vi "GetDigitalInputVals.vi"(8 "error in (no error)":errorcluster, 11 "SerialPortRef":T1) -> (0 "error out":errorcluster, 2 "32 bit array":bool[](array[boolean]), 3 "SerialPortRef 2":T1)   [LabVIEW 2015]
uses:
  <vilib>/Rock Robotics/WPI/SerialPort/WPI_SerialPortRef.ctl
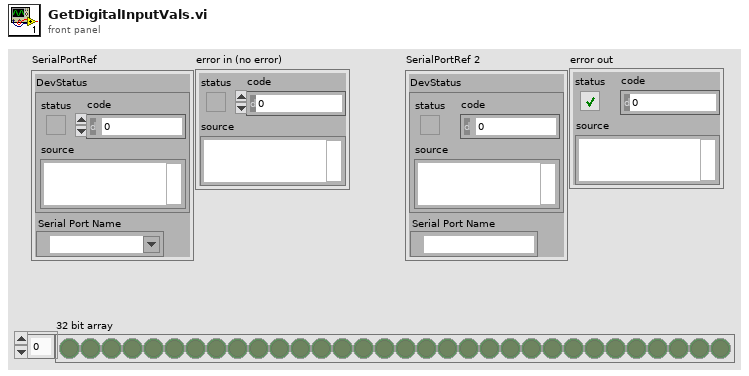
[diagram p1: front panel]
types:
  T1 = typedef "WPI_SerialPortRef.ctl" = cluster{"DevStatus":errorcluster, "Serial Port Name":refnum<visa-resource-name>}
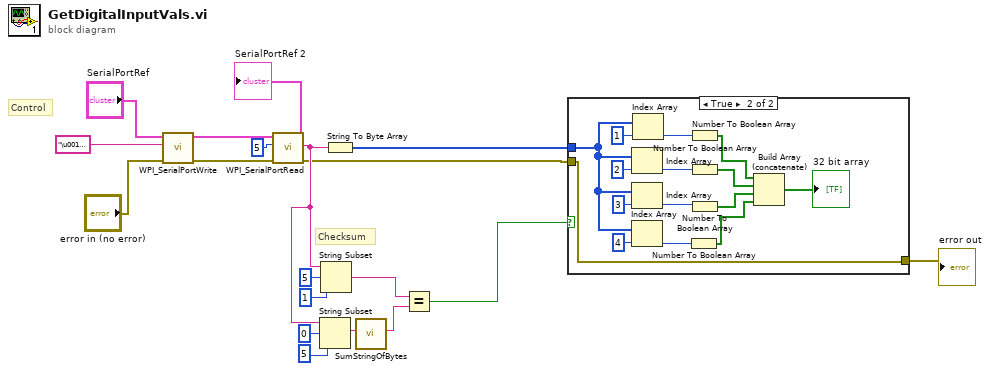
[diagram p0: block diagram]
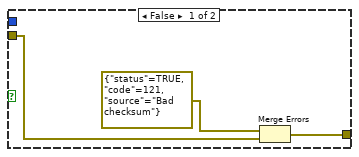
[diagram p2: hidden frame]
diagram:
  # "Checksum"
  # "Control"
  n1 = call <vilib>:"WPI_SerialPortWrite.vi"("error in (no error)"="error in (no error)", "Buffer"="\u0010\u0010", "SerialPortRef"="SerialPortRef") -> ("error out"=w15:errorcluster, "SerialPortRef"=w16:T1)  [unwired: 6 in, 1 out]
  n2 = call <vilib>:"WPI_SerialPortRead.vi"("error in (no error)"=w15, "Num Bytes to Read"=u32 5, "SerialPortRef"=w16) -> ("error out"=w3:errorcluster, "Buffer"=w9:string, "SerialPortRef"=→"SerialPortRef 2":T1)  [unwired: 6 in]
  n3 = String Subset(string=w9, offset (0)=0, length (rest)=5 ("length (rest)")) -> (substring=w6:string)
  n4 = String Subset(string=w9, offset (0)=5, length (rest)=1 ("length (rest)")) -> (substring=w5:string)
  n5 = String To Byte Array(string=w9) -> (unsigned byte array=w12:u8[])
  n6 = call "SumStringOfBytes.vi"("String Of Bytes"=w6) -> ("SumAsString"=w4:string)  [unwired: 10 in]
  n7 = Equal?(x=w5, y=w4) -> (x = y?=w2:bool)
  n8 = case shown="True" w2 {
    tunnel: w12 -> [_ w24]
    tunnel: w3 -> [w21 w23]
    tunnel: [w20 w23] -> w1
    frame False {
      n9 = Merge Errors(errorcluster {"status"=TRUE, "code"=121, "source"="Bad checksum"} ("error in"), w21) -> (w20:errorcluster)
    }
    frame True {
      n10 = Index Array(array=w24, index=2) -> (element=w30:u8)
      n11 = Index Array(array=w24, index=3) -> (element=w31:u8)
      n12 = Index Array(array=w24, index=4) -> (element=w32:u8)
      n13 = Index Array(array=w24, index=1) -> (element=w33:u8)
      n14 = Number To Boolean Array(number=w32) -> (Boolean array=w26:bool[])
      n15 = Number To Boolean Array(number=w33) -> (Boolean array=w29:bool[])
      n16 = Number To Boolean Array(number=w30) -> (Boolean array=w28:bool[])
      n17 = Number To Boolean Array(number=w31) -> (Boolean array=w27:bool[])
      n18 = Build Array (concatenate)(w29, w28, w27, w26) -> (→"32 bit array":bool[])
    }
  }
  "error out" <- w1
